vi "front_panel.vi"() -> ()   [LabVIEW 2019]
panel:
  in  "Units":i32(ring)=2 items=["µL/min", "µL/hr", "mL/min", "mL/hr"]
  in  "Flow rate":dbl=5.0 format="%.3f"
  in  "Dispense Volume (mL)":dbl=0.1 format="%_6f"
  in  "Syringe Inside Diameter":dbl=19.58 min=0.1 max=50.0 step=0.01 format="%#_4g"
  out "Output":string[][](array[string])
  in  "Column":i16[](array[numeric])
  in  "Row":i16[](array[numeric])=[4, 4]
  in  "Excel Filename":string="test.xls"
  in  "Sampling Interval (ms)":i32=5000
  out "RPP Reading":T1(array[cluster])
  in  "VISA Resource Names":refnum<visa-resource-name>[](array[refnum])
  in  "Lower Threshold":dbl=75.0
  in  "Upper Threshold":dbl=125.0
  # "For help, refer to the documentation at:\nhttps://github.com/pl9ed/RPP-Control/blob/master/README.md"
  # "Date                                                              Time                                                             Read Value                                                    Lower Threshold                                         Upper Threshold                                          Action                                                          Volume Dispensed"
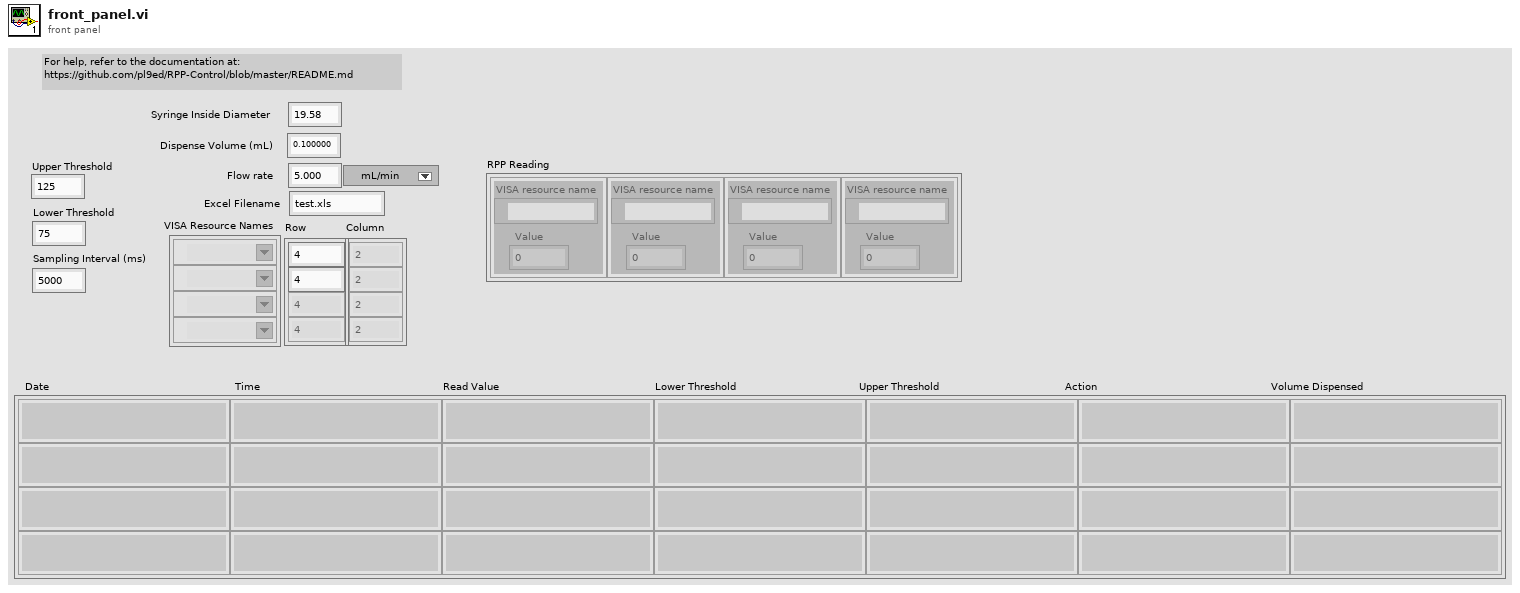
[diagram p1: front panel]
types:
  T1 = cluster{"Value":dbl, "VISA resource name":refnum<visa-resource-name>}[]
  T2 = cluster{"Read Value":dbl, "VISA resource name":refnum<visa-resource-name>}[]
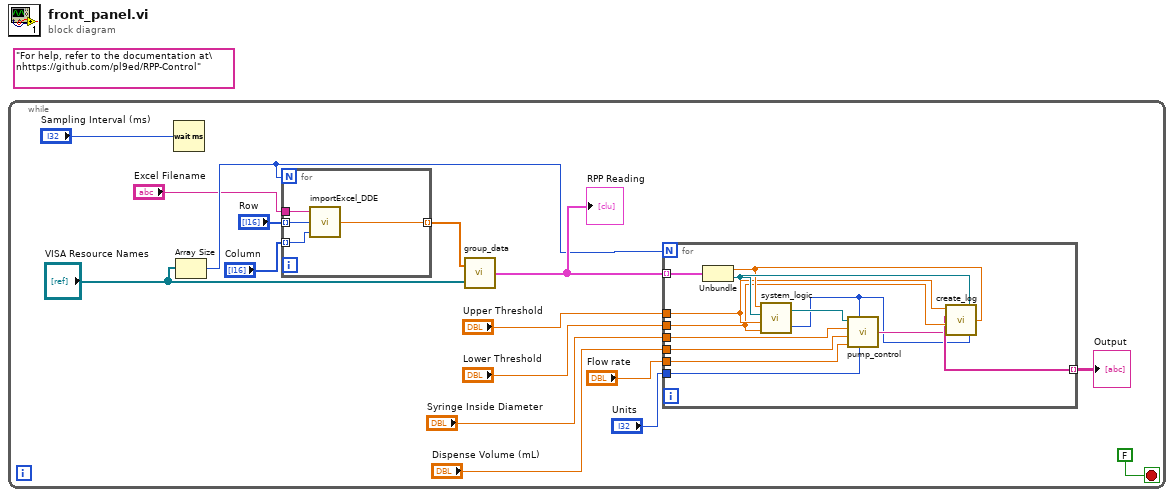
[diagram p0: block diagram]
diagram:
  (unwired) "For help, refer to the documentation at\nhttps://github.com/pl9ed/RPP-Control" ("String")
  n1 = while {
    stop <- FALSE stop-if-true
    n2 = Wait (ms)(milliseconds to wait="Sampling Interval (ms)") -> ()  [unwired: 1 out]
    n3 = Array Size(array="VISA Resource Names") -> (size(s)=w9:i32)
    n4 = for {
      N: w9 -> [_]
      tunnel: [w20] -> w10 mode=indexing
      tunnel: "Excel Filename" -> [w19]
      tunnel: "Column" -> [w18] mode=indexing
      tunnel: "Row" -> [w17] mode=indexing
      n5 = call "importExcel_DDE.vi"("COLUMN"=w18, "ROW"=w17, "Filename"=w19) -> ("Value"=w20:dbl)
    }
    n6 = call "group_data.vi"("VISA Resource Names"="VISA Resource Names", "Input Values"=w10) -> ("Grouped Data"=w16:T2)
    "RPP Reading" <- w16
    n7 = for {
      N: w9 -> [_]
      tunnel: w16 -> [w33] mode=indexing
      tunnel: "Upper Threshold" -> [w30]
      tunnel: "Lower Threshold" -> [w29]
      tunnel: [w28] -> w11 mode=indexing
      tunnel: "Dispense Volume (mL)" -> [w24]
      tunnel: "Units" -> [w23]
      tunnel: "Flow rate" -> [w22]
      tunnel: "Syringe Inside Diameter" -> [w21]
      n8 = Unbundle(w33) -> ("Read Value"=w31:dbl, "VISA resource name"=w32:refnum<visa-resource-name>)
      n9 = call "system_logic.vi"("Lower Threshold"=w29, "Upper Threshold"=w30, "VISA Name in"=w32, "Value"=w31) -> ("Action"=w25:u16, "VISA Name out"=w27:refnum<visa-resource-name>)
      n10 = call "pump_control.vi"("VISA resource name"=w27, "Direction"=w25, "Syringe Inside Diameter (19.58 mm)\nIf diameter is upper than 14.00 mm : Volume units are mL\nIf diameter is lower than 14.00 mm : Volume units are µL"=w21, "Dispense Volume (mL)"=w24, "Units"=w23, "Flow rate"=w22) -> ("Volume Dispensed"=w26:string)  [unwired: 2 out]
      n11 = call "create_log.vi"("Action"=w25, "Read Value"=w31, "VISA resource name"=w32, "Volume Dispensed"=w26, "Lower Threshold"=w29, "Upper Threshold"=w30) -> ("Output Array"=w28:string[])
    }
    "Output" <- w11
  }
